vi "Cycle_Diag_Table_Read.vi"(7 "ERD Data In":cluster{"ERD Number":u16, "Data":string}[](array[cluster]) {"ERD Number" format="%.0x"}, 11 "error in (no error)":errorcluster) -> (2 "Cycle Buffer Status":T2, 3 "Diag Cycle String Out":string[][](array[string]), 8 "Cycle  Diag Array Out":T1[](array[typedef]), 15 "error out":errorcluster)   [LabVIEW 2016]
uses:
  Type Definitions/2015 Program/Cycle_Diag_Buffer_Status.ctl
  Type Definitions/2015 Program/Cycle_Diag.ctl
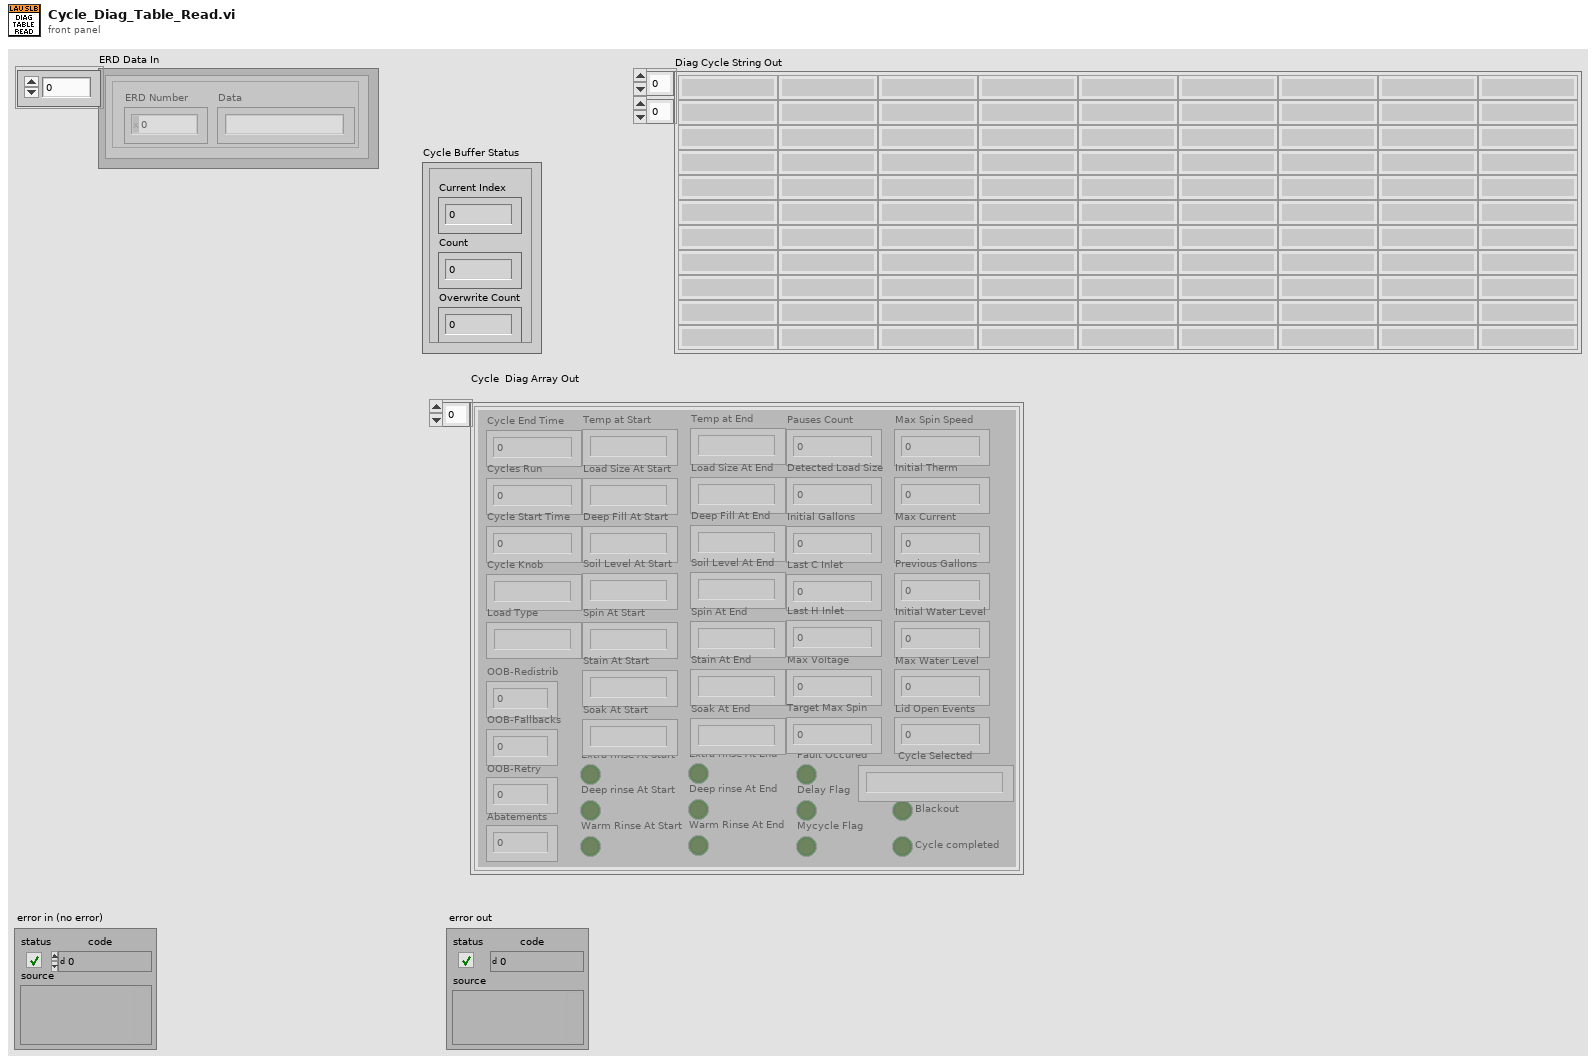
[diagram p1: front panel]
types:
  T1 = typedef "Cycle_Diag.ctl" = cluster{"Cycle End Time":u32, "Cycles Run":u32, "Cycle Start Time":u32, "Cycle Knob":string, "Load Type":string, "OOB-Redistrib":u8, "OOB-Fallbacks":u8, "OOB-Retry":u8, "Temp at Start":string, "Load Size At Start":string, "Deep Fill At Start":string, "Soil Level At Start":string, "Spin At Start":string, "Extra rinse At Start":bool, "Deep rinse At Start":bool, "Stain At Start":string, "Soak At Start":string, "Warm Rinse At Start":bool, "Temp at End":string, "Load Size At End":string, "Deep Fill At End":string, "Soil Level At End":string, "Spin At End":string, "Extra rinse At End":bool, "Deep rinse At End":bool, "Stain At End":string, "Soak At End":string, "Warm Rinse At End":bool, "Pauses Count":u8, "Fault Occured":bool, "Delay Flag":bool, "Mycycle Flag":bool, "Blackout":bool, "Cycle completed":bool, "Detected Load Size":dbl, "Initial Gallons":dbl, "Last C Inlet ":dbl, "Max Voltage":dbl, "Target Max Spin":u16, "Max Spin Speed":u16, "Initial Therm":dbl, "Max Current":dbl, "Previous Gallons":dbl, "Initial Water Level":dbl, "Max Water Level":dbl, "Abatements ":u8, "Lid Open Events":u8, "Cycle Selected":string, "Last H Inlet ":dbl}
  T2 = typedef "Cycle_Diag_Buffer_Status.ctl" = cluster{"Current Index":u16, "Count":u16, "Overwrite Count":u16}
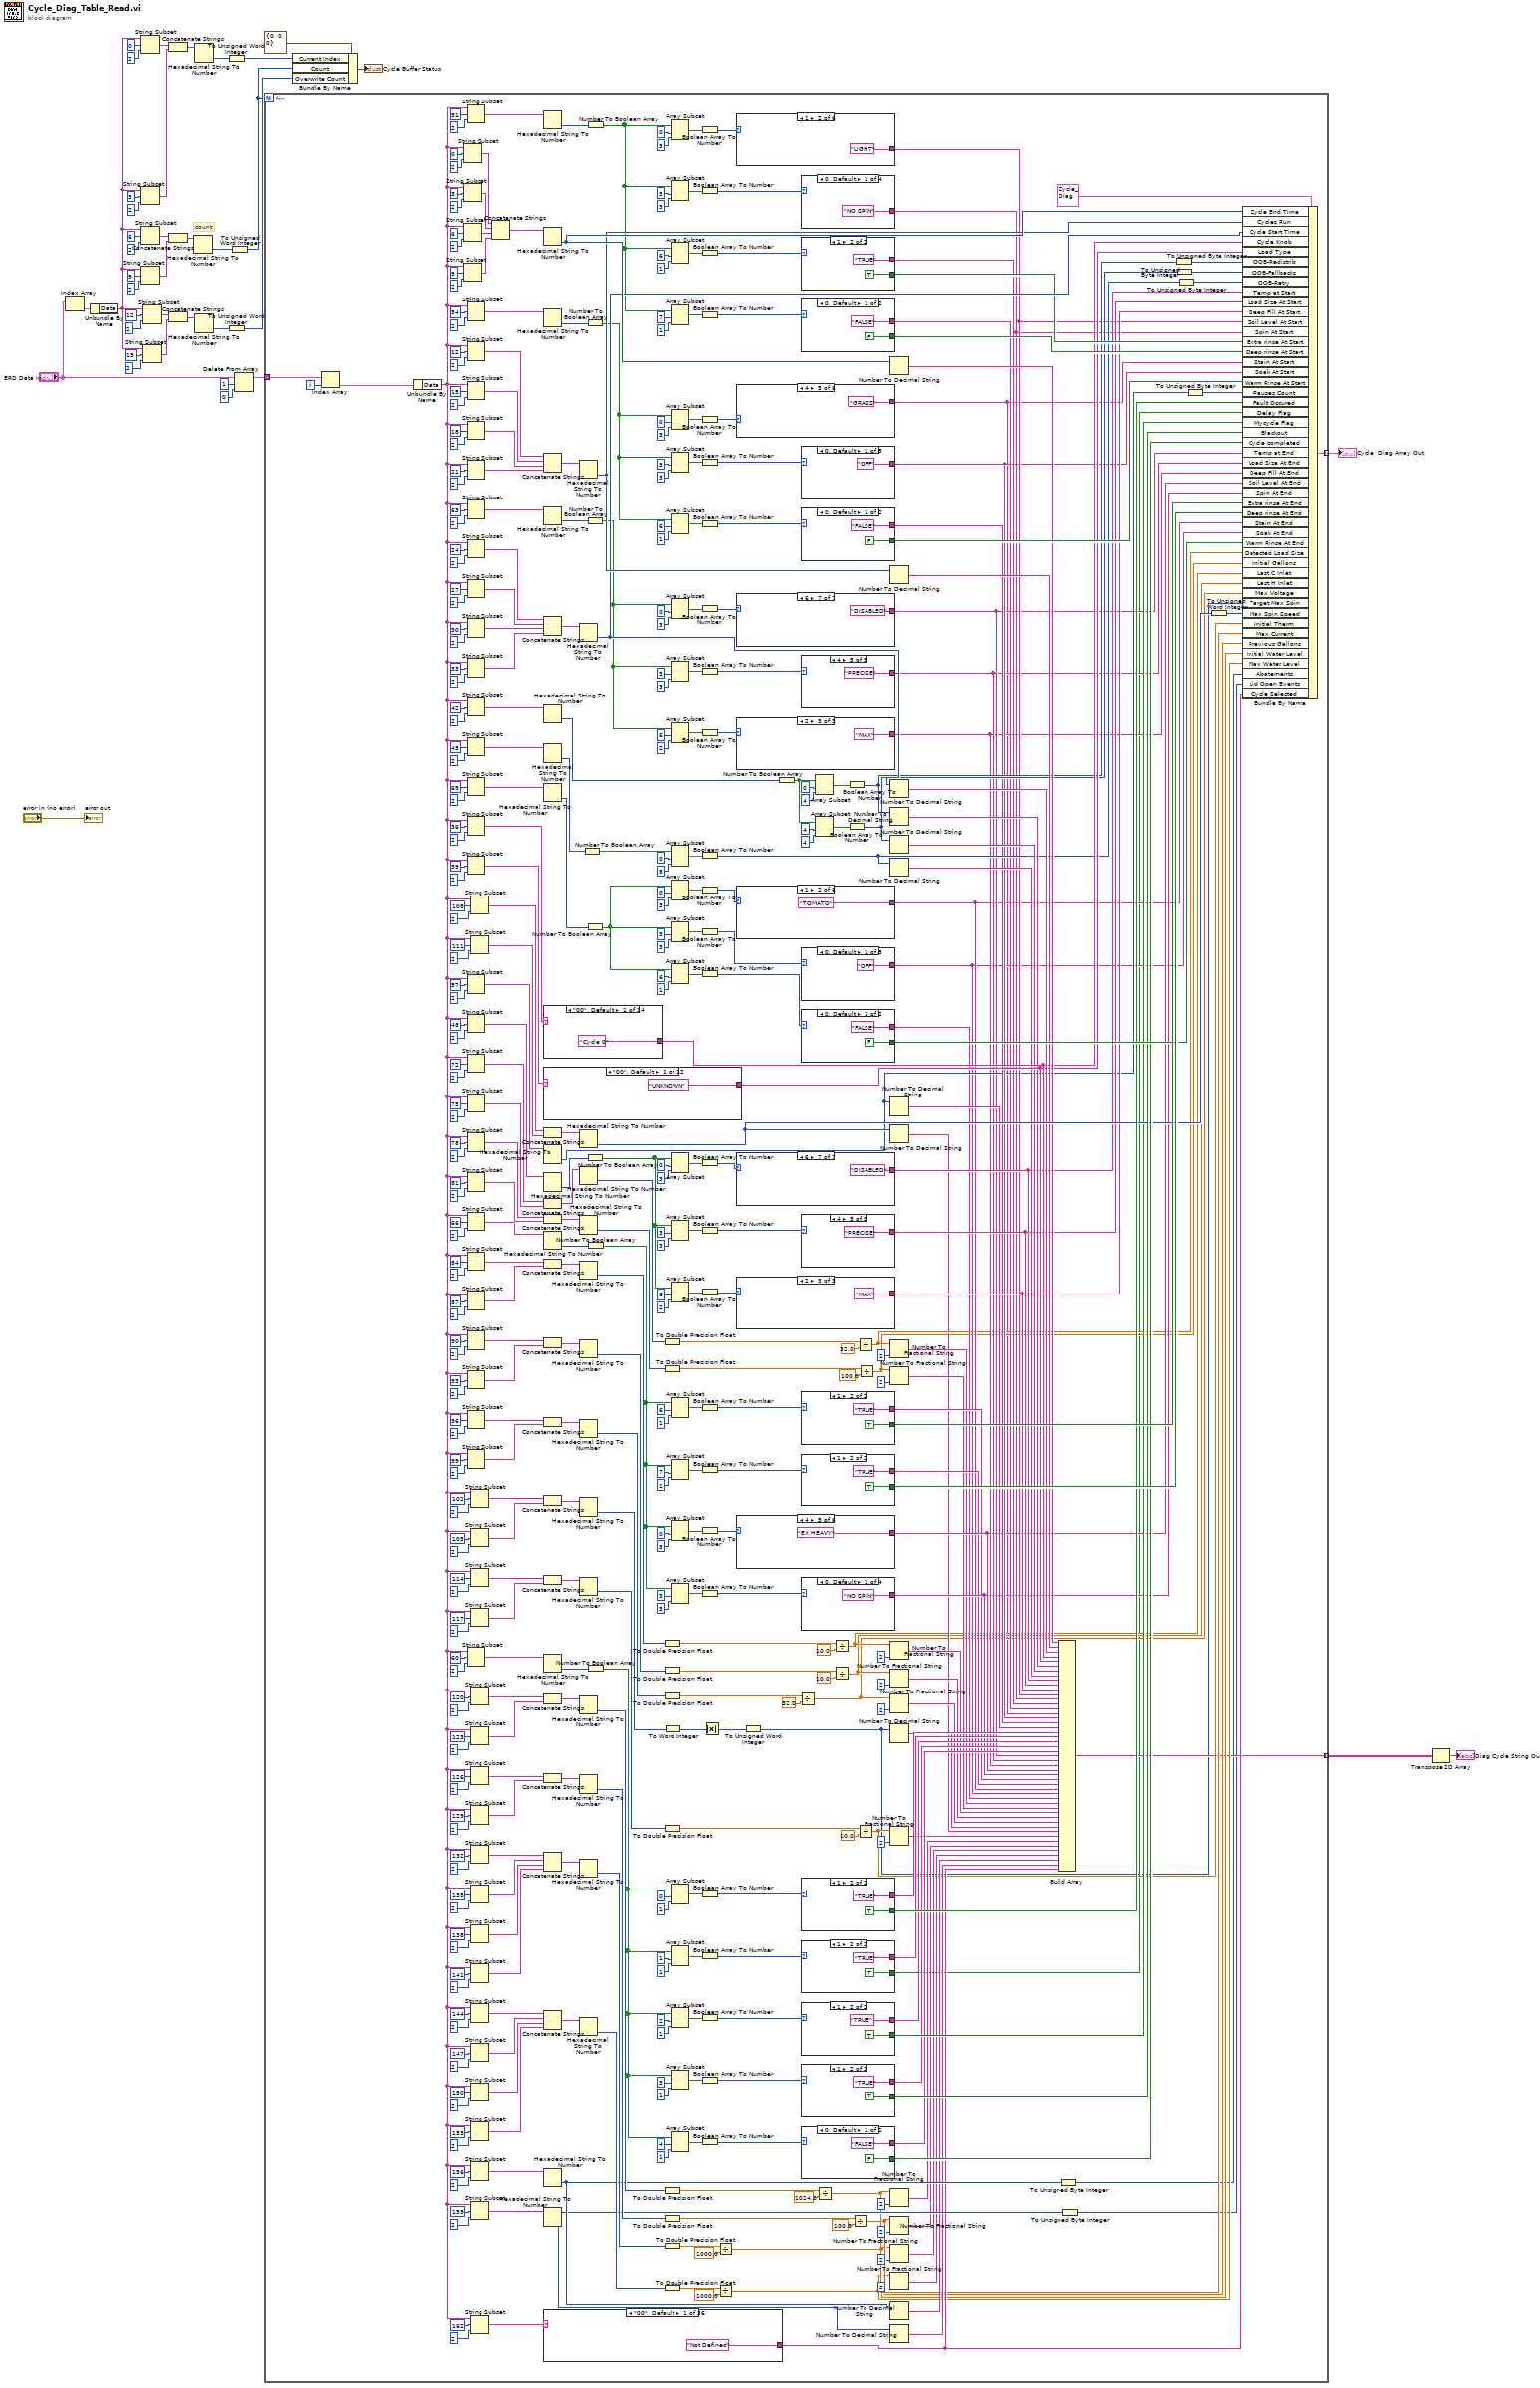
[diagram p0: block diagram]
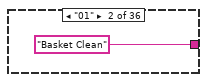
[diagram p2: hidden frame]
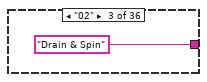
[diagram p3: hidden frame]
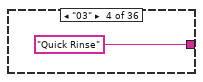
[diagram p4: hidden frame]
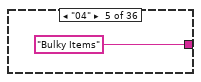
[diagram p5: hidden frame]
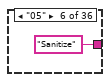
[diagram p6: hidden frame]
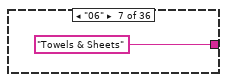
[diagram p7: hidden frame]
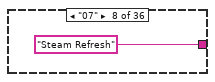
[diagram p8: hidden frame]
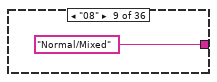
[diagram p9: hidden frame]
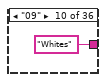
[diagram p10: hidden frame]
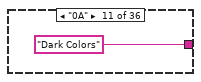
[diagram p11: hidden frame]
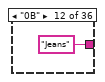
[diagram p12: hidden frame]
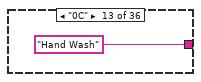
[diagram p13: hidden frame]
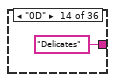
[diagram p14: hidden frame]
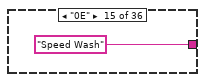
[diagram p15: hidden frame]
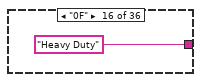
[diagram p16: hidden frame]
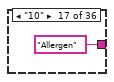
[diagram p17: hidden frame]
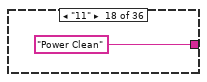
[diagram p18: hidden frame]
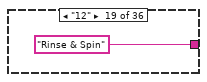
[diagram p19: hidden frame]
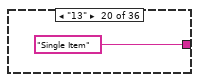
[diagram p20: hidden frame]
diagram:
  # "count"
  n1 = Index Array(array="ERD Data In") -> (element=w32:cluster{"ERD Number":u16, "Data":string})  [unwired: 1 in]
  n2 = Unbundle By Name(w32) -> ("Data"=w12:string)
  n3 = String Subset(string=w12, offset (0)=0, length (rest)=2 ("length (rest)")) -> (substring=w21:string)
  n4 = String Subset(string=w12, offset (0)=3, length (rest)=2 ("length (rest)")) -> (substring=w22:string)
  n5 = String Subset(string=w12, offset (0)=6, length (rest)=2 ("length (rest)")) -> (substring=w36:string)
  n6 = String Subset(string=w12, offset (0)=9, length (rest)=2 ("length (rest)")) -> (substring=w35:string)
  n7 = String Subset(string=w12, offset (0)=12, length (rest)=2 ("length (rest)")) -> (substring=w23:string)
  n8 = String Subset(string=w12, offset (0)=15, length (rest)=2 ("length (rest)")) -> (substring=w24:string)
  n9 = Concatenate Strings(w21, w22) -> (w25:string)
  n10 = Concatenate Strings(w36, w35) -> (w34:string)
  n11 = Concatenate Strings(w23, w24) -> (w26:string)
  n12 = Hexadecimal String To Number(string=w34) -> (number=w33:u32)  [unwired: 2 in, 1 out]
  n13 = Hexadecimal String To Number(string=w25) -> (number=w27:u32)  [unwired: 2 in, 1 out]
  n14 = Hexadecimal String To Number(string=w26) -> (number=w28:u32)  [unwired: 2 in, 1 out]
  n15 = To Unsigned Word Integer(number=w27) -> (unsigned 16bit integer=w29:u16)
  n16 = To Unsigned Word Integer(number=w28) -> (unsigned 16bit integer=w30:u16)
  n17 = To Unsigned Word Integer(number=w33) -> (unsigned 16bit integer=w11:u16)
  n18 = Delete From Array(array="ERD Data In", length=1, index=0) -> (array with subset deleted=w8:cluster{"ERD Number":u16, "Data":string}[])  [unwired: 1 out]
  n19 = for {
    N: w11 -> [_]
    tunnel: w8 -> [w238]
    tunnel: [w234] -> w4 mode=indexing
    tunnel: [w171] -> w3 mode=indexing
    i -> [w237]
    n20 = Index Array(array=w238, index=w237) -> (element=w236:cluster{"ERD Number":u16, "Data":string})
    n21 = Unbundle By Name(w236) -> ("Data"=w235:string)
    n22 = String Subset(string=w235, offset (0)=0, length (rest)=2 ("length (rest)")) -> (substring=w452:string)
    n23 = String Subset(string=w235, offset (0)=3, length (rest)=2 ("length (rest)")) -> (substring=w451:string)
    n24 = String Subset(string=w235, offset (0)=6, length (rest)=2 ("length (rest)")) -> (substring=w450:string)
    n25 = String Subset(string=w235, offset (0)=9, length (rest)=2 ("length (rest)")) -> (substring=w449:string)
    n26 = String Subset(string=w235, offset (0)=51, length (rest)=2 ("length (rest)")) -> (substring=w149:string)
    n27 = String Subset(string=w235, offset (0)=54, length (rest)=2 ("length (rest)")) -> (substring=w133:string)
    n28 = String Subset(string=w235, offset (0)=12, length (rest)=2 ("length (rest)")) -> (substring=w446:string)
    n29 = String Subset(string=w235, offset (0)=15, length (rest)=2 ("length (rest)")) -> (substring=w445:string)
    n30 = String Subset(string=w235, offset (0)=18, length (rest)=2 ("length (rest)")) -> (substring=w444:string)
    n31 = String Subset(string=w235, offset (0)=21, length (rest)=2 ("length (rest)")) -> (substring=w443:string)
    n32 = String Subset(string=w235, offset (0)=63, length (rest)=2 ("length (rest)")) -> (substring=w120:string)
    n33 = String Subset(string=w235, offset (0)=24, length (rest)=2 ("length (rest)")) -> (substring=w440:string)
    n34 = String Subset(string=w235, offset (0)=27, length (rest)=2 ("length (rest)")) -> (substring=w439:string)
    n35 = String Subset(string=w235, offset (0)=30, length (rest)=2 ("length (rest)")) -> (substring=w438:string)
    n36 = String Subset(string=w235, offset (0)=33, length (rest)=2 ("length (rest)")) -> (substring=w437:string)
    n37 = String Subset(string=w235, offset (0)=42, length (rest)=2 ("length (rest)")) -> (substring=w89:string)
    n38 = String Subset(string=w235, offset (0)=45, length (rest)=2 ("length (rest)")) -> (substring=w80:string)
    n39 = String Subset(string=w235, offset (0)=69, length (rest)=2 ("length (rest)")) -> (substring=w93:string)
    n40 = String Subset(string=w235, offset (0)=36, length (rest)=2 ("length (rest)")) -> (substring=w434:string)
    n41 = String Subset(string=w235, offset (0)=39, length (rest)=2 ("length (rest)")) -> (substring=w433:string)
    n42 = String Subset(string=w235, offset (0)=57, length (rest)=2 ("length (rest)")) -> (substring=w391:string)
    n43 = String Subset(string=w235, offset (0)=48, length (rest)=2 ("length (rest)")) -> (substring=w168:string)
    n44 = String Subset(string=w235, offset (0)=72, length (rest)=2 ("length (rest)")) -> (substring=w375:string)
    n45 = String Subset(string=w235, offset (0)=75 ("offset"), length (rest)=u32 2 ("default (0 U32)")) -> (substring=w372:string)
    n46 = String Subset(string=w235, offset (0)=78, length (rest)=2 ("length (rest)")) -> (substring=w367:string)
    n47 = String Subset(string=w235, offset (0)=81, length (rest)=2 ("length (rest)")) -> (substring=w366:string)
    n48 = String Subset(string=w235, offset (0)=66, length (rest)=2 ("length (rest)")) -> (substring=w106:string)
    n49 = String Subset(string=w235, offset (0)=84, length (rest)=2 ("length (rest)")) -> (substring=w356:string)
    n50 = String Subset(string=w235, offset (0)=87, length (rest)=2 ("length (rest)")) -> (substring=w355:string)
    n51 = String Subset(string=w235, offset (0)=90, length (rest)=2 ("length (rest)")) -> (substring=w350:string)
    n52 = String Subset(string=w235, offset (0)=93, length (rest)=2 ("length (rest)")) -> (substring=w349:string)
    n53 = String Subset(string=w235, offset (0)=96, length (rest)=2 ("length (rest)")) -> (substring=w340:string)
    n54 = String Subset(string=w235, offset (0)=99, length (rest)=2 ("length (rest)")) -> (substring=w339:string)
    n55 = String Subset(string=w235, offset (0)=60, length (rest)=2 ("length (rest)")) -> (substring=w390:string)
    n56 = String Subset(string=w235, offset (0)=108, length (rest)=2 ("length (rest)")) -> (substring=w327:string)
    n57 = String Subset(string=w235, offset (0)=111, length (rest)=2 ("length (rest)")) -> (substring=w326:string)
    n58 = String Subset(string=w235, offset (0)=102, length (rest)=2 ("length (rest)")) -> (substring=w330:string)
    n59 = String Subset(string=w235, offset (0)=105, length (rest)=2 ("length (rest)")) -> (substring=w329:string)
    n60 = String Subset(string=w235, offset (0)=114, length (rest)=2 ("length (rest)")) -> (substring=w315:string)
    n61 = String Subset(string=w235, offset (0)=117, length (rest)=2 ("length (rest)")) -> (substring=w314:string)
    n62 = String Subset(string=w235, offset (0)=120, length (rest)=2 ("length (rest)")) -> (substring=w305:string)
    n63 = String Subset(string=w235, offset (0)=123, length (rest)=2 ("length (rest)")) -> (substring=w304:string)
    n64 = String Subset(string=w235, offset (0)=126, length (rest)=2 ("length (rest)")) -> (substring=w295:string)
    n65 = String Subset(string=w235, offset (0)=129, length (rest)=2 ("length (rest)")) -> (substring=w294:string)
    n66 = String Subset(string=w235, offset (0)=132, length (rest)=2 ("length (rest)")) -> (substring=w285:string)
    n67 = String Subset(string=w235, offset (0)=135, length (rest)=2 ("length (rest)")) -> (substring=w284:string)
    n68 = String Subset(string=w235, offset (0)=138, length (rest)=2 ("length (rest)")) -> (substring=w254:string)
    n69 = String Subset(string=w235, offset (0)=141, length (rest)=2 ("length (rest)")) -> (substring=w253:string)
    n70 = String Subset(string=w235, offset (0)=144, length (rest)=2 ("length (rest)")) -> (substring=w279:string)
    n71 = String Subset(string=w235, offset (0)=147, length (rest)=2 ("length (rest)")) -> (substring=w278:string)
    n72 = String Subset(string=w235, offset (0)=150, length (rest)=2 ("length (rest)")) -> (substring=w248:string)
    n73 = String Subset(string=w235, offset (0)=153, length (rest)=2 ("length (rest)")) -> (substring=w247:string)
    n74 = String Subset(string=w235, offset (0)=156, length (rest)=2 ("length (rest)")) -> (substring=w259:string)
    n75 = String Subset(string=w235, offset (0)=159, length (rest)=2 ("length (rest)")) -> (substring=w258:string)
    n76 = String Subset(string=w235, offset (0)=162, length (rest)=2 ("length (rest)")) -> (substring=w255:string)
    n77 = Concatenate Strings(w452, w451, w450, w449) -> (w448:string)
    n78 = Hexadecimal String To Number(string=w149) -> (number=w156:u32)  [unwired: 2 in, 1 out]
    n79 = Hexadecimal String To Number(string=w448) -> (number=w447:u32)  [unwired: 2 in, 1 out]
    n80 = Hexadecimal String To Number(string=w133) -> (number=w141:u32)  [unwired: 2 in, 1 out]
    n81 = Concatenate Strings(w446, w445, w444, w443) -> (w442:string)
    n82 = Hexadecimal String To Number(string=w120) -> (number=w128:u32)  [unwired: 2 in, 1 out]
    n83 = Concatenate Strings(w440, w439, w438, w437) -> (w436:string)
    n84 = Hexadecimal String To Number(string=w89) -> (number=w88:u32)  [unwired: 2 in, 1 out]
    n85 = Hexadecimal String To Number(string=w80) -> (number=w79:u32)  [unwired: 2 in, 1 out]
    n86 = Hexadecimal String To Number(string=w93) -> (number=w101:u32)  [unwired: 2 in, 1 out]
    n87 = case shown="\"00\", Default" w434 {
      tunnel: ["Cycle 0" "Cycle 1" "Cycle 2" "Cycle 3" "Cycle 4" "Cycle 5" "Cycle 6" "Cycle 7" "Cycle 8" "Cycle 9" "Cycle 10" "Cycle 11" "Cycle 12" "Cycle 13"] -> w230
      frame "00", Default {
      }
      frame "01" {
      }
      frame "02" {
      }
      frame "03" {
      }
      frame "04" {
      }
      frame "05" {
      }
      frame "06" {
      }
      frame "07" {
      }
      frame "08" {
      }
      frame "09" {
      }
      frame "0A" {
      }
      frame "0B" {
      }
      frame "0C" {
      }
      frame "0D" {
      }
    }
    n88 = case shown="\"00\", Default" w433 {
      tunnel: ["UNKNOWN" "COTTON" "SYNTHETIC" "MIXED" "WET" "LOW FLOW" "SMALL" "MEDIUM" "LARGE" "SUPER" "SUPER PLUS" "MAX"] -> w229
      frame "00", Default {
      }
      frame "01" {
      }
      frame "02" {
      }
      frame "03" {
      }
      frame "04" {
      }
      frame "05" {
      }
      frame "06" {
      }
      frame "07" {
      }
      frame "08" {
      }
      frame "09" {
      }
      frame "0A" {
      }
      frame "0B" {
      }
    }
    n89 = Concatenate Strings(w327, w326) -> (w325:string)
    n90 = Hexadecimal String To Number(string=w391) -> (number=w213:u32)  [unwired: 2 in, 1 out]
    n91 = Hexadecimal String To Number(string=w168) -> (number=w167:u32)  [unwired: 2 in, 1 out]
    n92 = Concatenate Strings(w375, w372) -> (w371:string)
    n93 = Concatenate Strings(w367, w366) -> (w365:string)
    n94 = Hexadecimal String To Number(string=w106) -> (number=w116:u32)  [unwired: 2 in, 1 out]
    n95 = Concatenate Strings(w356, w355) -> (w354:string)
    n96 = Concatenate Strings(w350, w349) -> (w348:string)
    n97 = Concatenate Strings(w340, w339) -> (w338:string)
    n98 = Concatenate Strings(w330, w329) -> (w328:string)
    n99 = Concatenate Strings(w315, w314) -> (w313:string)
    n100 = Hexadecimal String To Number(string=w390) -> (number=w389:u32)  [unwired: 2 in, 1 out]
    n101 = Concatenate Strings(w305, w304) -> (w303:string)
    n102 = Concatenate Strings(w295, w294) -> (w293:string)
    n103 = Concatenate Strings(w285, w284, w254, w253) -> (w283:string)
    n104 = Concatenate Strings(w279, w278, w248, w247) -> (w277:string)
    n105 = Hexadecimal String To Number(string=w259) -> (number=w257:u32)  [unwired: 2 in, 1 out]
    n106 = Hexadecimal String To Number(string=w258) -> (number=w256:u32)  [unwired: 2 in, 1 out]
    n107 = case shown="\"00\", Default" w255 {
      tunnel: ["Not Defined" "Basket Clean" "Drain & Spin" "Quick Rinse" "Bulky Items" "Sanitize" "Towels & Sheets" "Steam Refresh" "Normal/Mixed" "Whites" "Dark Colors" "Jeans" "Hand Wash" "Delicates" "Speed Wash" "Heavy Duty" "Allergen" "Power Clean" "Rinse & Spin" "Single Item" "Colors" "Cold Wash" "Cottons" "Easy Care" "Active Wear" "Timed Dry" "Dewrinkle" "Air Fluff" "Steam Refresh" "Steam Dewrinkle" "Speed Dry" "Mixed" "Quick Dry" "Casuals" "Warm Up" "Energy Saver"] -> w180
      frame "00", Default {
      }
      frame "01" {
      }
      frame "02" {
      }
      frame "03" {
      }
      frame "04" {
      }
      frame "05" {
      }
      frame "06" {
      }
      frame "07" {
      }
      frame "08" {
      }
      frame "09" {
      }
      frame "0A" {
      }
      frame "0B" {
      }
      frame "0C" {
      }
      frame "0D" {
      }
      frame "0E" {
      }
      frame "0F" {
      }
      frame "10" {
      }
      frame "11" {
      }
      frame "12" {
      }
      frame "13" {
      }
      frame "14" {
      }
      frame "15" {
      }
      frame "80" {
      }
      frame "81" {
      }
      frame "82" {
      }
      frame "83" {
      }
      frame "84" {
      }
      frame "85" {
      }
      frame "86" {
      }
      frame "87" {
      }
      frame "88" {
      }
      frame "89" {
      }
      frame "8A" {
      }
      frame "8B" {
      }
      frame "8C" {
      }
      frame "8D" {
      }
    }
    n108 = Hexadecimal String To Number(string=w442) -> (number=w441:u32)  [unwired: 2 in, 1 out]
    n109 = Hexadecimal String To Number(string=w436) -> (number=w435:u32)  [unwired: 2 in, 1 out]
    n110 = Hexadecimal String To Number(string=w325) -> (number=w324:u32)  [unwired: 2 in, 1 out]
    n111 = Hexadecimal String To Number(string=w371) -> (number=w378:u32)  [unwired: 2 in, 1 out]
    n112 = Hexadecimal String To Number(string=w365) -> (number=w364:u32)  [unwired: 2 in, 1 out]
    n113 = Hexadecimal String To Number(string=w354) -> (number=w353:u32)  [unwired: 2 in, 1 out]
    n114 = Hexadecimal String To Number(string=w348) -> (number=w347:u32)  [unwired: 2 in, 1 out]
    n115 = Hexadecimal String To Number(string=w338) -> (number=w337:u32)  [unwired: 2 in, 1 out]
    n116 = Hexadecimal String To Number(string=w328) -> (number=w240:u32)  [unwired: 2 in, 1 out]
    n117 = Hexadecimal String To Number(string=w313) -> (number=w312:u32)  [unwired: 2 in, 1 out]
    n118 = Hexadecimal String To Number(string=w303) -> (number=w302:u32)  [unwired: 2 in, 1 out]
    n119 = Hexadecimal String To Number(string=w293) -> (number=w292:u32)  [unwired: 2 in, 1 out]
    n120 = Hexadecimal String To Number(string=w283) -> (number=w282:u32)  [unwired: 2 in, 1 out]
    n121 = Hexadecimal String To Number(string=w277) -> (number=w276:u32)  [unwired: 2 in, 1 out]
    n122 = Number To Boolean Array(number=w79) -> (Boolean array=w78:bool[])
    n123 = Number To Boolean Array(number=w141) -> (Boolean array=w140:bool[])
    n124 = Number To Boolean Array(number=w128) -> (Boolean array=w127:bool[])
    n125 = Number To Boolean Array(number=w101) -> (Boolean array=w100:bool[])
    n126 = Number To Boolean Array(number=w167) -> (Boolean array=w166:bool[])
    n127 = Number To Boolean Array(number=w156) -> (Boolean array=w148:bool[])
    n128 = Number To Boolean Array(number=w116) -> (Boolean array=w109:bool[])
    n129 = Number To Boolean Array(number=w389) -> (Boolean array=w64:bool[])
    n130 = To Double Precision Float(number=w378) -> (double precision float=w377:dbl)
    n131 = To Double Precision Float(number=w364) -> (double precision float=w363:dbl)
    n132 = To Double Precision Float(number=w353) -> (double precision float=w352:dbl)
    n133 = To Double Precision Float(number=w347) -> (double precision float=w346:dbl)
    n134 = To Double Precision Float(number=w337) -> (double precision float=w336:dbl)
    n135 = To Word Integer(number=w240) -> (16bit integer=w242:i16)
    n136 = To Double Precision Float(number=w312) -> (double precision float=w311:dbl)
    n137 = To Double Precision Float(number=w302) -> (double precision float=w301:dbl)
    n138 = To Double Precision Float(number=w292) -> (double precision float=w291:dbl)
    n139 = To Double Precision Float(number=w282) -> (double precision float=w281:dbl)
    n140 = To Double Precision Float(number=w276) -> (double precision float=w275:dbl)
    n141 = Array Subset(array=w148, index=0, length=3) -> (w145:bool[])
    n142 = Array Subset(array=w148, index=3, length=3) -> (w144:bool[])
    n143 = Array Subset(array=w148, index=6, length=1) -> (w143:bool[])
    n144 = Array Subset(array=w148, index=7, length=1) -> (w142:bool[])
    n145 = Array Subset(array=w140, index=0, length=3) -> (w131:bool[])
    n146 = Array Subset(array=w140, index=3, length=3) -> (w130:bool[])
    n147 = Array Subset(array=w140, index=6, length=1) -> (w129:bool[])
    n148 = Array Subset(array=w127, index=0, length=3) -> (w119:bool[])
    n149 = Array Subset(array=w127, index=3, length=3) -> (w118:bool[])
    n150 = Array Subset(array=w127, index=6, length=2) -> (w117:bool[])
    n151 = Array Subset(array=w78, index=0, length=8) -> (w75:bool[])
    n152 = Array Subset(array=w100, index=0, length=3) -> (w92:bool[])
    n153 = Array Subset(array=w100, index=3, length=3) -> (w91:bool[])
    n154 = Array Subset(array=w100, index=6, length=1) -> (w90:bool[])
    n155 = Array Subset(array=w166, index=0, length=3) -> (w159:bool[])
    n156 = Array Subset(array=w166, index=3, length=3) -> (w158:bool[])
    n157 = Array Subset(array=w166, index=6, length=2) -> (w157:bool[])
    n158 = Array Subset(array=w109, index=6, length=1) -> (w103:bool[])
    n159 = Array Subset(array=w109, index=7, length=1) -> (w102:bool[])
    n160 = Array Subset(array=w109, index=0, length=3) -> (w105:bool[])
    n161 = Array Subset(array=w109, index=3, length=3) -> (w104:bool[])
    n162 = Array Subset(array=w64, index=0, length=1) -> (w63:bool[])
    n163 = Array Subset(array=w64, index=1, length=1) -> (w61:bool[])
    n164 = Array Subset(array=w64, index=2, length=1) -> (w60:bool[])
    n165 = Array Subset(array=w64, index=3, length=1) -> (w59:bool[])
    n166 = Array Subset(array=w64, index=4, length=1) -> (w58:bool[])
    n167 = Boolean Array To Number(Boolean array=w145) -> (number=w424:u32)
    n168 = Boolean Array To Number(Boolean array=w144) -> (number=w423:u32)
    n169 = Boolean Array To Number(Boolean array=w143) -> (number=w422:u32)
    n170 = Boolean Array To Number(Boolean array=w142) -> (number=w421:u32)
    n171 = Boolean Array To Number(Boolean array=w131) -> (number=w418:u32)
    n172 = Boolean Array To Number(Boolean array=w130) -> (number=w417:u32)
    n173 = Boolean Array To Number(Boolean array=w129) -> (number=w416:u32)
    n174 = Boolean Array To Number(Boolean array=w119) -> (number=w408:u32)
    n175 = Boolean Array To Number(Boolean array=w118) -> (number=w407:u32)
    n176 = Boolean Array To Number(Boolean array=w117) -> (number=w406:u32)
    n177 = Boolean Array To Number(Boolean array=w75) -> (number=w223:u32)
    n178 = Boolean Array To Number(Boolean array=w92) -> (number=w401:u32)
    n179 = Boolean Array To Number(Boolean array=w91) -> (number=w400:u32)
    n180 = Boolean Array To Number(Boolean array=w90) -> (number=w399:u32)
    n181 = Boolean Array To Number(Boolean array=w159) -> (number=w239:u32)
    n182 = Boolean Array To Number(Boolean array=w158) -> (number=w426:u32)
    n183 = Boolean Array To Number(Boolean array=w157) -> (number=w425:u32)
    n184 = Boolean Array To Number(Boolean array=w103) -> (number=w403:u32)
    n185 = Boolean Array To Number(Boolean array=w102) -> (number=w402:u32)
    n186 = Boolean Array To Number(Boolean array=w105) -> (number=w405:u32)
    n187 = Boolean Array To Number(Boolean array=w104) -> (number=w404:u32)
    n188 = Boolean Array To Number(Boolean array=w63) -> (number=w388:u32)
    n189 = Boolean Array To Number(Boolean array=w61) -> (number=w387:u32)
    n190 = Boolean Array To Number(Boolean array=w60) -> (number=w386:u32)
    n191 = Boolean Array To Number(Boolean array=w59) -> (number=w385:u32)
    n192 = Boolean Array To Number(Boolean array=w58) -> (number=w384:u32)
    n193 = Absolute Value(x=w242) -> (abs(x)=w241:i16)
    n194 = Divide(x=w281, y=1000.0) -> (x/y=w173:dbl)
    n195 = Divide(x=w275, y=1000.0) -> (x/y=w172:dbl)
    n196 = case shown="1" w424 {
      tunnel: ["EXTRA LIGHT" "LIGHT" "NORMAL" "HEAVY" "EX HEAVY" "DISABLED"] -> w219
      frame 0, Default {
      }
      frame 1 {
      }
      frame 2 {
      }
      frame 3 {
      }
      frame 4 {
      }
      frame 5 {
      }
    }
    n197 = case shown="4" w418 {
      tunnel: ["OFF" "TOMATO" "WINE" "BLOOD" "GRASS" "DIRT"] -> w132
      frame 0, Default {
      }
      frame 1 {
      }
      frame 2 {
      }
      frame 3 {
      }
      frame 4 {
      }
      frame 5 {
      }
    }
    n198 = case shown="6" w408 {
      tunnel: ["TAP COLD" "COLD" "COOL" "COLORS" "WARM" "HOT" "DISABLED"] -> w205
      frame 0, Default {
      }
      frame 1 {
      }
      frame 2 {
      }
      frame 3 {
      }
      frame 4 {
      }
      frame 5 {
      }
      frame 6 {
      }
    }
    n199 = case shown="2" w406 {
      tunnel: ["OFF" "INCREMENTAL" "MAX"] -> w203
      frame 0, Default {
      }
      frame 1 {
      }
      frame 2 {
      }
    }
    n200 = case shown="1" w401 {
      tunnel: ["OFF" "TOMATO" "WINE" "BLOOD" "GRASS" "DIRT"] -> w198
      frame 0, Default {
      }
      frame 1 {
      }
      frame 2 {
      }
      frame 3 {
      }
      frame 4 {
      }
      frame 5 {
      }
    }
    n201 = case shown="6" w239 {
      tunnel: ["TAP COLD" "COLD" "COOL" "COLORS" "WARM" "HOT" "DISABLED"] -> w222
      frame 0, Default {
      }
      frame 1 {
      }
      frame 2 {
      }
      frame 3 {
      }
      frame 4 {
      }
      frame 5 {
      }
      frame 6 {
      }
    }
    n202 = case shown="2" w425 {
      tunnel: ["OFF" "INCREMENTAL" "MAX"] -> w220
      frame 0, Default {
      }
      frame 1 {
      }
      frame 2 {
      }
    }
    n203 = case shown="4" w405 {
      tunnel: ["EXTRA LIGHT" "LIGHT" "NORMAL" "HEAVY" "EX HEAVY" "DISABLED"] -> w202
      frame 0, Default {
      }
      frame 1 {
      }
      frame 2 {
      }
      frame 3 {
      }
      frame 4 {
      }
      frame 5 {
      }
    }
    n204 = To Unsigned Word Integer(number=w241) -> (unsigned 16bit integer=w47:u16)
    n205 = Number To Boolean Array(number=w88) -> (Boolean array=w83:bool[])
    n206 = Divide(x=w336, y=32.0) -> (x/y=w177:dbl)
    n207 = case shown="0, Default" w423 {
      tunnel: ["NO SPIN" "NORMAL" "MORE" "MAX"] -> w218
      frame 0, Default {
      }
      frame 1 {
      }
      frame 2 {
      }
      frame 3 {
      }
    }
    n208 = case shown="1" w422 {
      tunnel: [FALSE TRUE] -> w420
      tunnel: ["FALSE" "TRUE"] -> w217
      frame 0, Default {
      }
      frame 1 {
      }
    }
    n209 = case shown="0, Default" w421 {
      tunnel: [FALSE TRUE] -> w419
      tunnel: ["FALSE" "TRUE"] -> w216
      frame 0, Default {
      }
      frame 1 {
      }
    }
    n210 = case shown="0, Default" w417 {
      tunnel: ["OFF" "15 MIN" "30 MIN" "60 MIN" "2 HOURS"] -> w215
      frame 0, Default {
      }
      frame 1 {
      }
      frame 2 {
      }
      frame 3 {
      }
      frame 4 {
      }
    }
    n211 = case shown="0, Default" w416 {
      tunnel: [FALSE TRUE] -> w415
      tunnel: ["FALSE" "TRUE"] -> w214
      frame 0, Default {
      }
      frame 1 {
      }
    }
    n212 = case shown="4" w407 {
      tunnel: ["SMALL" "MEDIUM" "LARGE" "SUPER" "PRECISE"] -> w204
      frame 0, Default {
      }
      frame 1 {
      }
      frame 2 {
      }
      frame 3 {
      }
      frame 4 {
      }
    }
    n213 = case shown="0, Default" w400 {
      tunnel: ["OFF" "15 MIN" "30 MIN" "60 MIN" "2 HOURS"] -> w197
      frame 0, Default {
      }
      frame 1 {
      }
      frame 2 {
      }
      frame 3 {
      }
      frame 4 {
      }
    }
    n214 = case shown="0, Default" w399 {
      tunnel: [FALSE TRUE] -> w396
      tunnel: ["FALSE" "TRUE"] -> w196
      frame 0, Default {
      }
      frame 1 {
      }
    }
    n215 = case shown="4" w426 {
      tunnel: ["SMALL" "MEDIUM" "LARGE" "SUPER" "PRECISE"] -> w221
      frame 0, Default {
      }
      frame 1 {
      }
      frame 2 {
      }
      frame 3 {
      }
      frame 4 {
      }
    }
    n216 = case shown="1" w403 {
      tunnel: [FALSE TRUE] -> w398
      tunnel: ["FALSE" "TRUE"] -> w200
      frame 0, Default {
      }
      frame 1 {
      }
    }
    n217 = case shown="1" w402 {
      tunnel: [FALSE TRUE] -> w397
      tunnel: ["FALSE" "TRUE"] -> w199
      frame 0, Default {
      }
      frame 1 {
      }
    }
    n218 = case shown="0, Default" w404 {
      tunnel: ["NO SPIN" "NORMAL" "MORE" "MAX"] -> w201
      frame 0, Default {
      }
      frame 1 {
      }
      frame 2 {
      }
      frame 3 {
      }
    }
    n219 = case shown="1" w388 {
      tunnel: [FALSE TRUE] -> w383
      tunnel: ["FALSE" "TRUE"] -> w210
      frame 0, Default {
      }
      frame 1 {
      }
    }
    n220 = case shown="1" w387 {
      tunnel: [FALSE TRUE] -> w62
      tunnel: ["FALSE" "TRUE"] -> w209
      frame 0, Default {
      }
      frame 1 {
      }
    }
    n221 = case shown="1" w386 {
      tunnel: [FALSE TRUE] -> w211
      tunnel: ["FALSE" "TRUE"] -> w208
      frame 0, Default {
      }
      frame 1 {
      }
    }
    n222 = case shown="1" w385 {
      tunnel: [FALSE TRUE] -> w382
      tunnel: ["FALSE" "TRUE"] -> w207
      frame 0, Default {
      }
      frame 1 {
      }
    }
    n223 = case shown="0, Default" w384 {
      tunnel: [FALSE TRUE] -> w381
      tunnel: ["FALSE" "TRUE"] -> w206
      frame 0, Default {
      }
      frame 1 {
      }
    }
    n224 = Array Subset(array=w83, index=0, length=4) -> (w82:bool[])
    n225 = Array Subset(array=w83, index=4, length=4) -> (w81:bool[])
    n226 = Divide(x=w301, y=1024.0) -> (x/y=w175:dbl)
    n227 = Divide(x=w352, y=10.0) -> (x/y=w179:dbl)
    n228 = Divide(x=w346, y=10.0) -> (x/y=w178:dbl)
    n229 = Boolean Array To Number(Boolean array=w82) -> (number=w228:u32)
    n230 = Boolean Array To Number(Boolean array=w81) -> (number=w226:u32)
    n231 = Divide(x=w291, y=100.0) -> (x/y=w174:dbl)
    n232 = Divide(x=w377, y=32.0) -> (x/y=w195:dbl)
    n233 = Divide(x=w311, y=10.0) -> (x/y=w176:dbl)
    n234 = Divide(x=w363, y=100.0) -> (x/y=w170:dbl)
    n235 = Number To Decimal String(number=w447) -> (decimal integer string=w233:string)  [unwired: 1 in]
    n236 = Number To Decimal String(number=w441) -> (decimal integer string=w232:string)  [unwired: 1 in]
    n237 = Number To Decimal String(number=w435) -> (decimal integer string=w231:string)  [unwired: 1 in]
    n238 = Number To Decimal String(number=w228) -> (decimal integer string=w227:string)  [unwired: 1 in]
    n239 = Number To Decimal String(number=w226) -> (decimal integer string=w225:string)  [unwired: 1 in]
    n240 = Number To Decimal String(number=w223) -> (decimal integer string=w224:string)  [unwired: 1 in]
    n241 = Number To Decimal String(number=w213) -> (decimal integer string=w212:string)  [unwired: 1 in]
    n242 = Number To Decimal String(number=w324) -> (decimal integer string=w188:string)  [unwired: 1 in]
    n243 = Number To Fractional String(number=w195, precision (6)=i16 2) -> (F-format string=w194:string)  [unwired: 2 in]
    n244 = Number To Fractional String(number=w170, precision (6)=i16 2) -> (F-format string=w193:string)  [unwired: 2 in]
    n245 = Number To Fractional String(number=w179, precision (6)=i16 2) -> (F-format string=w192:string)  [unwired: 2 in]
    n246 = Number To Fractional String(number=w178, precision (6)=i16 2) -> (F-format string=w191:string)  [unwired: 2 in]
    n247 = Number To Fractional String(number=w177, precision (6)=i16 2) -> (F-format string=w190:string)  [unwired: 2 in]
    n248 = Number To Decimal String(number=w47) -> (decimal integer string=w189:string)  [unwired: 1 in]
    n249 = Number To Fractional String(number=w176, precision (6)=i16 2) -> (F-format string=w187:string)  [unwired: 2 in]
    n250 = Number To Fractional String(number=w175, precision (6)=i16 2) -> (F-format string=w186:string)  [unwired: 2 in]
    n251 = Number To Fractional String(number=w174, precision (6)=i16 2) -> (F-format string=w185:string)  [unwired: 2 in]
    n252 = Number To Fractional String(number=w173, precision (6)=i16 2) -> (F-format string=w184:string)  [unwired: 2 in]
    n253 = Number To Fractional String(number=w172, precision (6)=i16 2) -> (F-format string=w183:string)  [unwired: 2 in]
    n254 = Number To Decimal String(number=w257) -> (decimal integer string=w182:string)  [unwired: 1 in]
    n255 = Number To Decimal String(number=w256) -> (decimal integer string=w181:string)  [unwired: 1 in]
    n256 = Build Array(w233, w232, w231, w230, w229, w227, w225, w224, w222, w221, w220, w219, w218, w217, w216, w132, w215, w214, w212, w210, w209, w208, w207, w206, w205, w204, w203, w202, w201, w200, w199, w198, w197, w196, w194, w193, w192, w191, w190, w189, w188, w187, w186, w185, w184, w183, w182, w181, w180) -> (w171:string[])
    n257 = To Unsigned Byte Integer(number=w257) -> (unsigned 8bit integer=w46:u8)
    n258 = To Unsigned Byte Integer(number=w256) -> (unsigned 8bit integer=w45:u8)
    n259 = To Unsigned Byte Integer(number=w228) -> (unsigned 8bit integer=w57:u8)
    n260 = To Unsigned Byte Integer(number=w226) -> (unsigned 8bit integer=w56:u8)
    n261 = To Unsigned Byte Integer(number=w223) -> (unsigned 8bit integer=w55:u8)
    n262 = To Unsigned Byte Integer(number=w213) -> (unsigned 8bit integer=w54:u8)
    n263 = To Unsigned Word Integer(number=w324) -> (unsigned 16bit integer=w48:u16)
    n264 = Bundle By Name(cluster=T1 {"Cycle End Time"=0, "Cycles Run"=0, "Cycle Start Time"=0, "Cycle Knob"="", "Load Type"="", "OOB-Redistrib"=0, "OOB-Fallbacks"=0, "OOB-Retry"=0, "Temp at Start"="", "Load Size At Start"="", "Deep Fill At Start"="", "Soil Level At Start"="", "Spin At Start"="", "Extra rinse At Start"=FALSE, "Deep rinse At Start"=FALSE, "Stain At Start"="", "Soak At Start"="", "Warm Rinse At Start"=FALSE, "Temp at End"="", "Load Size At End"="", "Deep Fill At End"="", "Soil Level At End"="", "Spin At End"="", "Extra rinse At End"=FALSE, "Deep rinse At End"=FALSE, "Stain At End"="", "Soak At End"="", "Warm Rinse At End"=FALSE, "Pauses Count"=0, "Fault Occured"=FALSE, "Delay Flag"=FALSE, "Mycycle Flag"=FALSE, "Blackout"=FALSE, "Cycle completed"=FALSE, "Detected Load Size"=0.0, "Initial Gallons"=0.0, "Last C Inlet "=0.0, "Max Voltage"=0.0, "Target Max Spin"=0, "Max Spin Speed"=0, "Initial Therm"=0.0, "Max Current"=0.0, "Previous Gallons"=0.0, "Initial Water Level"=0.0, "Max Water Level"=0.0, "Abatements "=0, "Lid Open Events"=0, "Cycle Selected"="", "Last H Inlet "=0.0} ("Cycle History Diagnostics"), "Cycle End Time"=w447, "Cycles Run"=w441, "Cycle Start Time"=w435, "Cycle Knob"=w230, "Load Type"=w229, "OOB-Redistrib"=w57, "OOB-Fallbacks"=w56, "OOB-Retry"=w55, "Temp at Start"=w222, "Load Size At Start"=w221, "Deep Fill At Start"=w220, "Soil Level At Start"=w219, "Spin At Start"=w218, "Extra rinse At Start"=w420, "Deep rinse At Start"=w419, "Stain At Start"=w132, "Soak At Start"=w215, "Warm Rinse At Start"=w415, "Pauses Count"=w54, "Fault Occured"=w383, "Delay Flag"=w62, "Mycycle Flag"=w211, "Blackout"=w382, "Cycle completed"=w381, "Temp at End"=w205, "Load Size At End"=w204, "Deep Fill At End"=w203, "Soil Level At End"=w202, "Spin At End"=w201, "Extra rinse At End"=w398, "Deep rinse At End"=w397, "Stain At End"=w198, "Soak At End"=w197, "Warm Rinse At End"=w396, "Detected Load Size"=w195, "Initial Gallons"=w170, "Last C Inlet"=w179, "Last H Inlet"=w178, "Max Voltage"=w177, "Target Max Spin"=w47, "Max Spin Speed"=w48, "Initial Therm"=w176, "Max Current"=w175, "Previous Gallons"=w174, "Initial Water Level"=w173, "Max Water Level"=w172, "Abatements"=w46, "Lid Open Events"=w45, "Cycle Selected"=w180) -> (w234:T1)
  }
  "Cycle  Diag Array Out" <- w4
  n265 = Bundle By Name(cluster=T2 {"Current Index"=0, "Count"=0, "Overwrite Count"=0} ("Cycle Buffer Status"), "Current Index"=w29, "Count"=w11, "Overwrite Count"=w30) -> (→"Cycle Buffer Status":T2)
  n266 = Transpose 2D Array(2D array=w3) -> (transposed array=→"Diag Cycle String Out":string[][])
  "error out" <- "error in (no error)"
